vi "CollorCellsInTableOnly copy.vi"(11 "Array":i64[][](array[numeric])) -> (3 "Matches Digits":string[][](table))   [LabVIEW 2023]
uses:
  <vilib>/Utility/file.llb/Read Delimited Spreadsheet (I64).vi
panel:
  in  "Tab Control":enum32{"Page 1", "Page 2"}(tab)
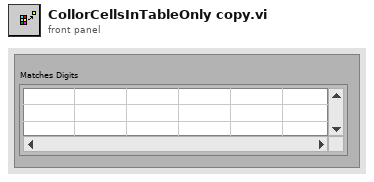
[diagram p1: front panel]
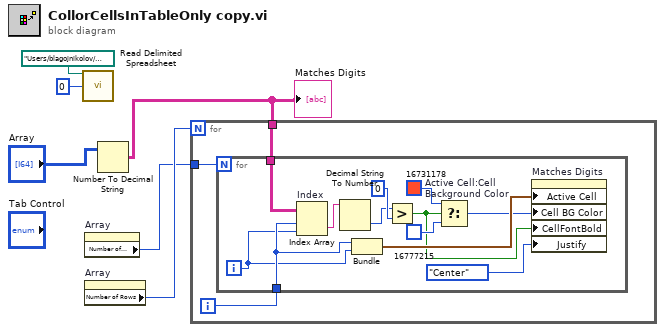
[diagram p0: block diagram]
diagram:
  n1 = call-poly <vilib>:"Read Delimited Spreadsheet.vi"("file path (dialog if empty)"=path "/Users/blagojnikolov/Desktop/@tmp/matches.txt", "start of read offset (chars.:0)"=0) -> ()  [unwired: 8 in, 6 out]
  n2 = property on="Array" class="Arr (strict)"() -> ("Number of Columns"=w5:u32)  [unwired: 2 in, 2 out]
  n3 = property on="Array" class="Arr (strict)"() -> ("Number of Rows"=w6:u32)  [unwired: 2 in, 2 out]
  n4 = Number To Decimal String(number="Array") -> (decimal integer string=w2:string[][])  [unwired: 1 in]
  "Matches Digits" <- w2
  n5 = for {
    N: w6 -> [_]
    tunnel: w5 -> [w9]
    tunnel: w2 -> [w8]
    i -> [w7]
    n6 = for {
      N: w9 -> [_]
      tunnel: w8 -> [w21]
      tunnel: w7 -> [w20]
      i -> [w19]
      w15 = u32 16731178  # Active Cell:Cell Background Color
      n7 = Index Array "Index"(array=w21, index (row)=w20, index (col)=w19) -> (element=w18:string)
      n8 = Decimal String To Number(string=w18) -> (number=w10:i32)  [unwired: 2 in, 1 out]
      n9 = Bundle(w20, w19) -> (w17:cluster{i32, i32})  [unwired: 1 in]
      n10 = Greater?(x=w10, y=0) -> (0:w11:bool)
      n11 = Select(t=w15, s=w11, f=u32 16777215 ("Active Cell:Cell Background Color")) -> (s? t:f=w14:u32)
      n12 = property on="Matches Digits" class="Tbl (strict)"("Active Cell"=w17, "Cell BG Color"=w14, "CellFontBold"=w11, "Justify"=enum16{"Left", "Center", "Right"}."Center" ("Active Cell:Cell Justification")) -> ()  [unwired: 2 in, 2 out]
    }
  }
